vi "Send Software Trigger.vi"(8 "error in (no error)":errorcluster, 11 "VISA resource name":refnum<visa-resource-name>) -> (0 "error out":errorcluster, 3 "VISA resource name out":refnum<visa-resource-name>)   [LabVIEW 2012, in "Agilent E364X Series.lvlib"]
doc: "This VI sends a command to trigger the power supply. Call this VI if you configure the power supply to respond to software triggers. If the power supply is not configured to respond to software triggers, this VI returns an error."
uses:
  Agilent E364X Series.lvlib
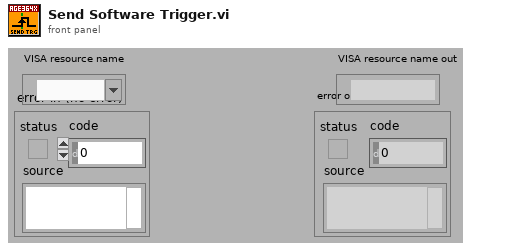
[diagram p1: front panel]
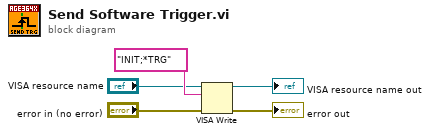
[diagram p0: block diagram]
diagram:
  n1 = VISA Write(VISA resource name="VISA resource name", write buffer="INIT;*TRG", error in (no error)="error in (no error)") -> (VISA resource name out=→"VISA resource name out":refnum<visa-resource-name>, error out=→"error out":errorcluster)  [unwired: 1 out]
